vi "close.vi"(8 "error in (no error)":errorcluster, 11 "Pixelfly in":refnum<class "Pixelfly.lvclass">) -> (0 "error out":errorcluster)   [LabVIEW 2009, in "Hardware.lvlib" / "Channels.lvlib" / "Pixelfly.lvclass"]
uses:
  Pixelfly.lvclass
  Pixelfly.lvclass/Pixelfly.ctl
panel:
  out "Buffer status":T1
  # "Status flags"
  # "Buffer errors"
  # "Memory usage"
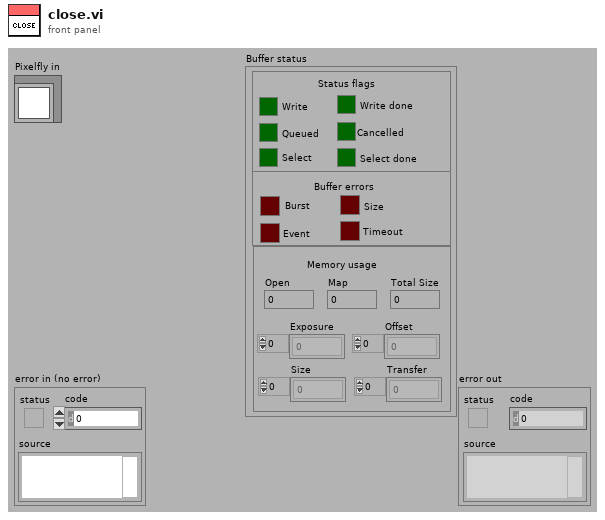
[diagram p1: front panel]
types:
  T1 = cluster{"Write":bool, "Write done":bool, "Queued":bool, "Cancelled":bool, "Select":bool, "Select done":bool, "Burst":bool, "Size":bool, "Event":bool, "Timeout":bool, "Open":i32, "Map":i32, "Exposure":i32[], "Offset":i32[], "Size":i32[], "Transfer":i32[], "Total Size":i32}
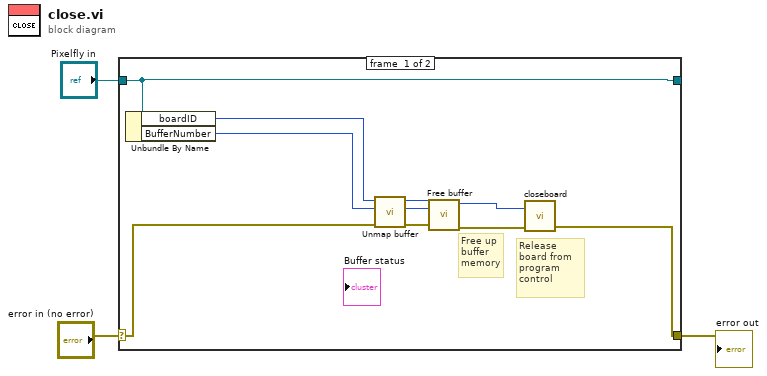
[diagram p0: block diagram]
diagram:
  n1 = case shown="No Error" "error in (no error)" {
    selector: "error in (no error)" -> [w5 w14]
    tunnel: [w11 w15] -> _
    tunnel: "Pixelfly in" -> [w11 w15]
    tunnel: [w10 w14] -> w1
    frame #0 {
      # "Release board from program control"
      # "Free up buffer memory"
      n2 = Unbundle By Name(w11) -> ("boardID"=w4:i32, "BufferNumber"=w6:i32)
      n3 = call <instrlib>:"Unmap buffer.vi"("error in (no error)"=w5, "Buffer in"=w6, "Handle in"=w4) -> ("error out"=w8:errorcluster, "Buffer number"=w7:i32, "Handle out"=w9:i32)  [unwired: 2 in]
      n4 = call <instrlib>:"Free buffer.vi"("error in (no error)"=w8, "Buffer in"=w7, "Handle in"=w9) -> ("error out"=w13:errorcluster, "Handle out"=w12:i32)  [unwired: 2 in, 1 out]
      n5 = call <instrlib>:"closeboard.vi"("Handle in"=w12, "error in (no error)"=w13) -> ("error out"=w10:errorcluster)  [unwired: 2 out]
    }
    frame #1 {
    }
  }
  "error out" <- w1
